vi "CycleXWithExtern.vi"(0 "Devices queue":refnum<queue>, 1 "Program only changes":bool, 5 "Program during MOT loading":bool, 7 "Igor Inform String":string[](array[string]), 9 "Additional wait time (s)":dbl, 11 "error in":errorcluster) -> (8 "error out":errorcluster)   [LabVIEW 2013]
uses:
  Device/Device.lvclass
  Master Device/Master Device.lvclass
  Globals/Total Time.vi
panel:
  out "Fatal Error":errorcluster caption="error out"
  # "Status and timing"
  # "Igor options"
  # "Hardware control"
  # "This option starts the pulse blaster and then programs the external devices.  If the MOT loading time is not long enough for this process to complete there will be problems."
  # "When set, this option only\nasks a device to program\nitself if it's hardware image\nhas actually changed."
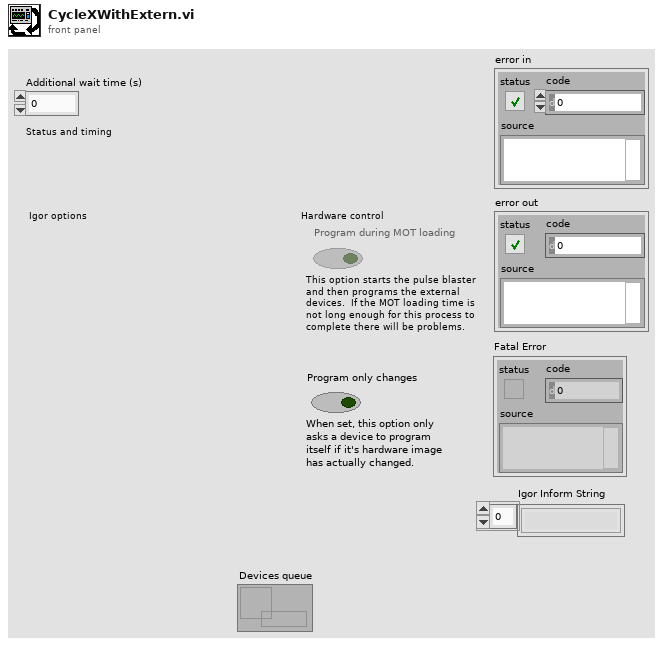
[diagram p1: front panel]
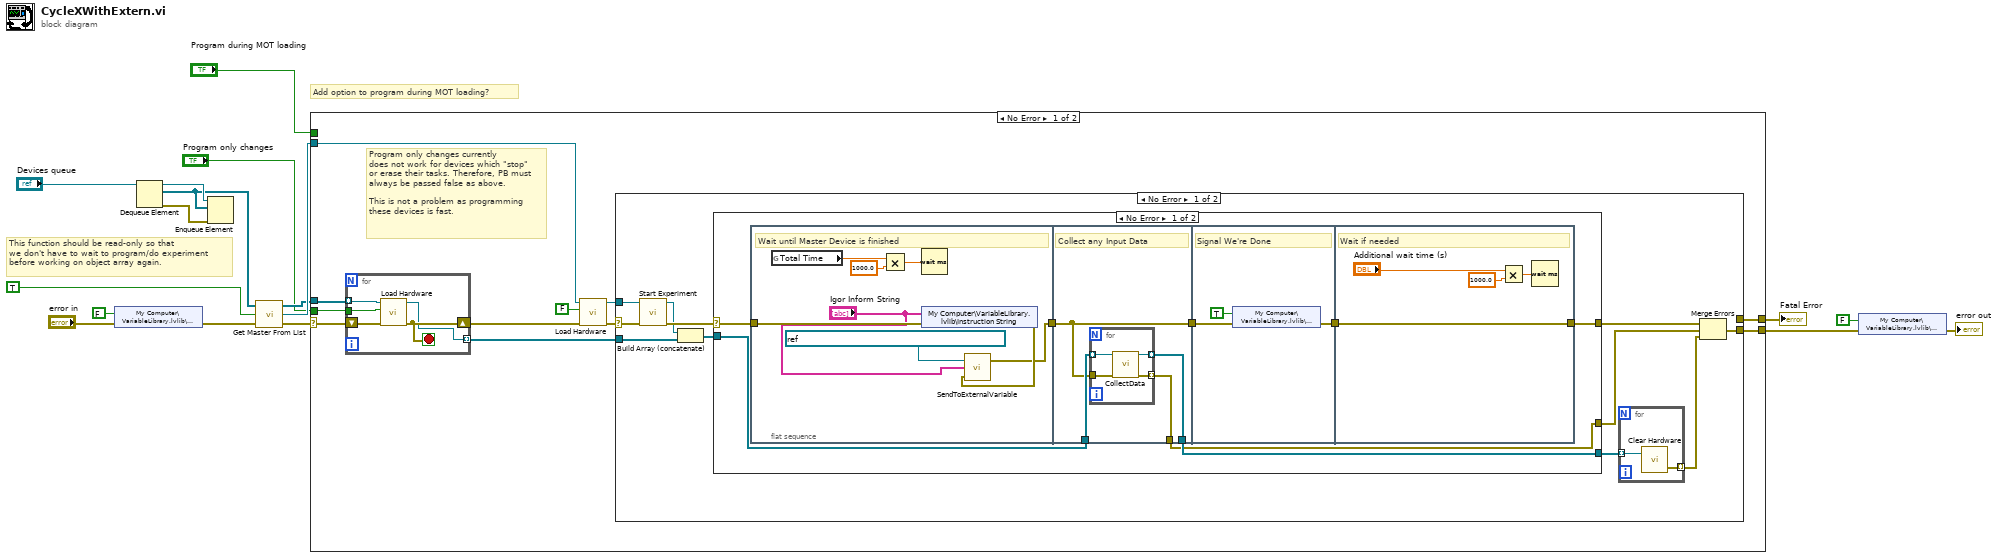
[diagram p0: block diagram]
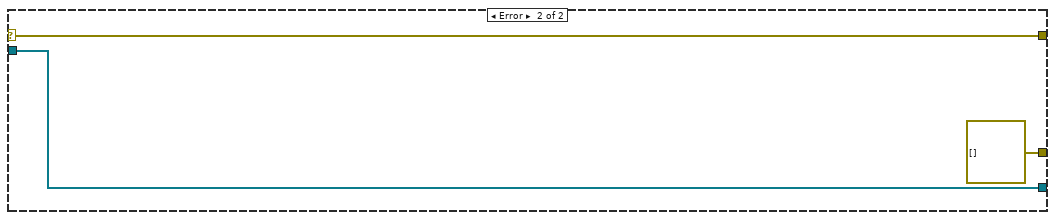
[diagram p2: hidden frame]
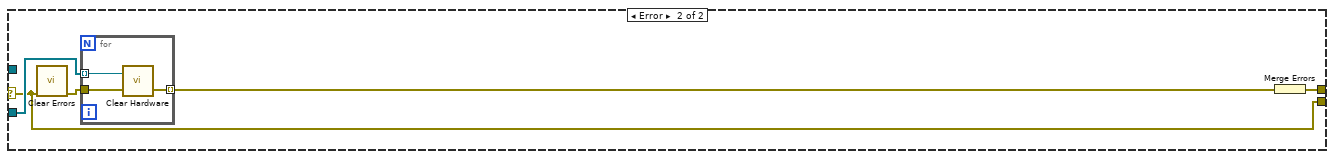
[diagram p3: hidden frame]
diagram:
  # "This function should be read-only so that \nwe don't have to wait to program/do experiment \nbefore working on object array again."
  # "Add option to program during MOT loading?"
  n1 = shared-variable "My Computer\\VariableLibrary.lvlib\\CycleDone"(FALSE ("CycleDone"), error in="error in") -> (error out=w9:errorcluster)
  n2 = Dequeue Element(queue="Devices queue") -> (queue out=w12:refnum<queue>, element=w11:refnum<class "Device.lvclass">[], error out=w10:errorcluster)  [unwired: 2 in, 1 out]
  n3 = Enqueue Element(queue=w12, element=w11, error in (no error)=w10) -> ()  [unwired: 1 in, 3 out]
  n4 = call "Get Master From List.vi"("error in"=w9, "Del From List?"=TRUE, "Device List in"=w11) -> ("error out"=w14:errorcluster, "Master Device"=w16:refnum<class "Master Device.lvclass">, "Device List out"=w15:refnum<class "Device.lvclass">[])
  n5 = case shown="No Error" w14 {
    selector: w14 -> [w23 w89]
    tunnel: w16 -> [w27 _]
    tunnel: w15 -> [w26 _]
    tunnel: [w22 w89] -> w5
    tunnel: "Program only changes" -> [w20 _]
    tunnel: [w18 _] -> w2
    tunnel: "Program during MOT loading" -> [_ _]
    frame No Error {
      # "Program only changes currently\ndoes not work for devices which \"stop\"\nor erase their tasks. Therefore, PB must\nalways be passed false as above.\n\nThis is not a problem as programming\nthese devices is fast."
      n6 = for {
        tunnel: w26 -> [w88] mode=indexing
        shift-right: [w86] -> w28
        shift-left: w23 -> [w87]
        tunnel: [w85] -> w25 mode=indexing
        tunnel: w20 -> [w84]
        stop <- w86 stop-if-true
        n7 = call-dynamic "Load Hardware.vi"("error in (no error)"=w87, "Program only changes"=w84, "Device in"=w88) -> ("error out"=w86:errorcluster, "Device out"=w85:refnum<class "Device.lvclass">)  [unwired: 7 in]
      }
      n8 = call-dynamic "Load Hardware.vi"("error in (no error)"=w28, "Program only changes"=FALSE, "Master Device in"=w27) -> ("error out"=w21:errorcluster, "Master Device out"=w24:refnum<class "Master Device.lvclass">)  [unwired: 7 in]
      n9 = case shown="No Error" w21 {
        selector: w21 -> [w36 w76]
        tunnel: w25 -> [w37 w80]
        tunnel: [w39 w76] -> w22
        tunnel: w24 -> [w38 _]
        tunnel: [_ w77] -> w18
        frame No Error {
          n10 = call-dynamic "Start Experiment.vi"("error in (no error)"=w36, "Master Device in"=w38) -> ("error out"=w35:errorcluster, "Master Device out"=w34:refnum<class "Master Device.lvclass">)  [unwired: 8 in]
          n11 = Build Array (concatenate)(w34, w37) -> (w33:refnum<class "Device.lvclass">[])
          n12 = case shown="No Error" w35 {
            selector: w35 -> [w47 w73]
            tunnel: [w45 w73] -> w31
            tunnel: w33 -> [w42 w72]
            tunnel: [w41 w72] -> w32
            tunnel: [w40 errorcluster[] []] -> w30
            frame No Error {
              n13 = flat-sequence {
                tunnel: w47 -> [w52]
                tunnel: [w48] -> w44
                tunnel: w44 -> [w57]
                tunnel: [w57] -> w43
                tunnel: w42 -> [w59]
                tunnel: [w58] -> w41
                tunnel: [w56] -> w40
                tunnel: w43 -> [w65]
                tunnel: [w64] -> w46
                tunnel: w46 -> [w67]
                tunnel: [w67] -> w45
                frame #0 {
                  # "Wait until Master Device is finished"
                  n14 = global read "Total Time.vi" "Total Time"() -> (w53:dbl)
                  n15 = Multiply(x=w53, y=1000.0) -> (x*y=w54:dbl)
                  n16 = Wait (ms)(milliseconds to wait=w54) -> ()  [unwired: 1 out]
                  n17 = shared-variable "My Computer\\VariableLibrary.lvlib\\Instruction String"("Igor Inform String", error in=w52) -> (error out=w49:errorcluster)
                  n18 = call "SendToExternalVariable.vi"("error In"=w49, "Igor Instruction String"="Igor Inform String", "Source of Data"=refnum<k21> "\\\\RbRyPc\\VariableLibrary\\Instruction String") -> ("error out"=w48:errorcluster)  [unwired: 1 in]
                }
                frame #1 {
                  # "Collect any Input Data"
                  n19 = for {
                    tunnel: w59 -> [w63] mode=indexing
                    tunnel: [w62] -> w58 mode=indexing
                    tunnel: w57 -> [w61]
                    tunnel: [w60] -> w56 mode=indexing
                    n20 = call-dynamic "CollectData.vi"("error in (no error)"=w61, "Device in"=w63) -> ("error out"=w60:errorcluster, "Device out"=w62:refnum<class "Device.lvclass">)  [unwired: 8 in]
                  }
                }
                frame #2 {
                  # "Signal We're Done"
                  n21 = shared-variable "My Computer\\VariableLibrary.lvlib\\CycleDone"(TRUE ("CycleDone"), error in=w65) -> (error out=w64:errorcluster)
                }
                frame #3 {
                  # "Wait if needed"
                  n22 = Multiply(x="Additional wait time (s)", y=1000.0) -> (x*y=w69:dbl)
                  n23 = Wait (ms)(milliseconds to wait=w69) -> ()  [unwired: 1 out]
                }
              }
            }
            frame Error {
            }
          }
          n24 = for {
            tunnel: w32 -> [w74] mode=indexing
            tunnel: [w75] -> w29 mode=indexing
            n25 = call-dynamic "Clear Hardware.vi"("Device in"=w74) -> ("error out"=w75:errorcluster)  [unwired: 1 in, 1 out]
          }
          n26 = Merge Errors(w31, w30, w29) -> (w39:errorcluster)
        }
        frame Error {
          n27 = call <vilib>:"Clear Errors.vi"("error in (no error)"=w76) -> ("error out"=w79:errorcluster)  [unwired: 6 in]
          n28 = for {
            tunnel: w80 -> [w82] mode=indexing
            tunnel: w79 -> [w83]
            tunnel: [w81] -> w78 mode=indexing
            n29 = call-dynamic "Clear Hardware.vi"("error in (no error)"=w83, "Device in"=w82) -> ("error out"=w81:errorcluster)  [unwired: 1 out]
          }
          n30 = Merge Errors(w78) -> (w77:errorcluster)
        }
      }
    }
    frame Error {
    }
  }
  "Fatal Error" <- w2
  n31 = shared-variable "My Computer\\VariableLibrary.lvlib\\CycleDone"(FALSE ("CycleDone"), error in=w5) -> (error out=→"error out":errorcluster)
